vi "Ethernet IP Custom Device Main Page.vi"(8 "error in (no error)":errorcluster, 11 "Node Ptr":T1 format="%.0x") -> (0 "error out":errorcluster)   [LabVIEW 2023, in "Ethernet IP Custom Device Custom Device.lvlib"]
uses:
  Ethernet IP Custom Device Custom Device.lvlib
  <vilib>/NI VeriStand/Custom Device API/Custom Device Item Ref.ctl
  <vilib>/NI VeriStand/Custom Device API/Custom Device Channel.ctl
  <vilib>/NI VeriStand/Custom Device API/Custom Device Channel Type.ctl
  Ethernet IP Global Strings.vi
  <vilib>/NI VeriStand/Custom Device API/Get Item Property (Path).vi
  <vilib>/NI VeriStand/Custom Device API/Get Item Property (I32).vi
  <vilib>/NI VeriStand/Custom Device API/Get Item Property (String).vi
  <vilib>/NI VeriStand/Custom Device API/Set Item Property (String).vi
  <vilib>/NI VeriStand/Custom Device API/Set Item Property (Path).vi
  Ethernet IP Global GUIDs.vi
  <vilib>/NI VeriStand/Custom Device API/Set Item Property (I32).vi
  <vilib>/NI VeriStand/Custom Device API/Custom Device API.lvlib
panel:
  in  "Import Assembly File":bool
  in  "Path to Assembly Import file":path
  in  "Import Selected File":bool
  in  "Path to L5K file":path
  in  "Update Rate (ms)":i32
  in  "Communication Timeout (ms)":i32
  in  "Logix Slot":u16
  in  "Backplane Port":u16
  in  "PLC Address (IP Address)":string
  in  "Header":cluster{"Section Name":string}={"Section Name"="Custom Device Item Settings"}
  in  "Description":string
  in  "Name":string
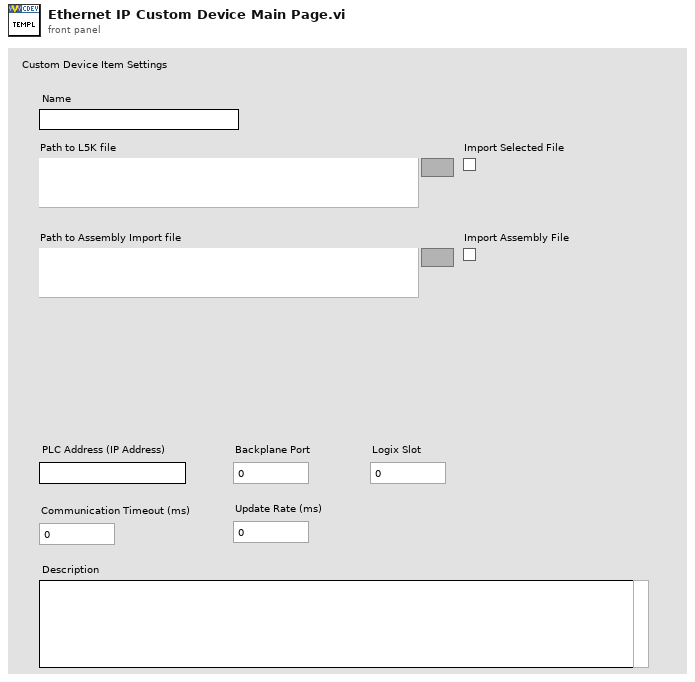
[diagram p1: front panel]
types:
  T1 = typedef "Custom Device API.lvlib/Custom Device Item Ref.ctl" = u64
  T2 = enum8{"Enabled", "Disabled", "Disabled and Grayed Out"}
  T3 = typedef "Custom Device API.lvlib/Custom Device Item Info.ctl" = cluster{"Name":string, "Is Channel":bool, "GUID":string, "Is Waveform":bool}
  T4 = typedef "Custom Device API.lvlib/Custom Device Channel.ctl" = cluster{"Type":T5, "Units":string, "Default Value":dbl, "Faultable":bool, "Scalable":bool}
  T5 = typedef "Custom Device API.lvlib/Custom Device Channel Type.ctl" = enum16{"Input", "Output"}
  T6 = typedef "Custom Device API.lvlib/Custom Device Commands.ctl" = enum16{"Default", "Item renamed", "Shutdown", "Dynamic button pressed"}
  T7 = typedef "Ethernet IP Custom Device Custom Device.lvlib/L5K Internal Data.ctl" = cluster{"L5K Entire String":string, "L5K Extractred String Array":string[], "IP address from CommPath":string, "Configured Tags":T8[], "Data String Array":string[], "Unconfigured Tags":T8[], "# Tags":i32}
  T8 = typedef "Ethernet IP Custom Device Custom Device.lvlib/L5K Tag.ctl" = cluster{"Tag Name":string, "Data Type":T9, "Data Type String":string, "Array Size":i32, "Description":string, "Input?":bool, "Channel Name":string}
  T9 = typedef "Ethernet IP Custom Device Custom Device.lvlib/L5K Data Types.ctl" = enum16{"SINT", "INT", "DINT", "REAL", "BOOL"}
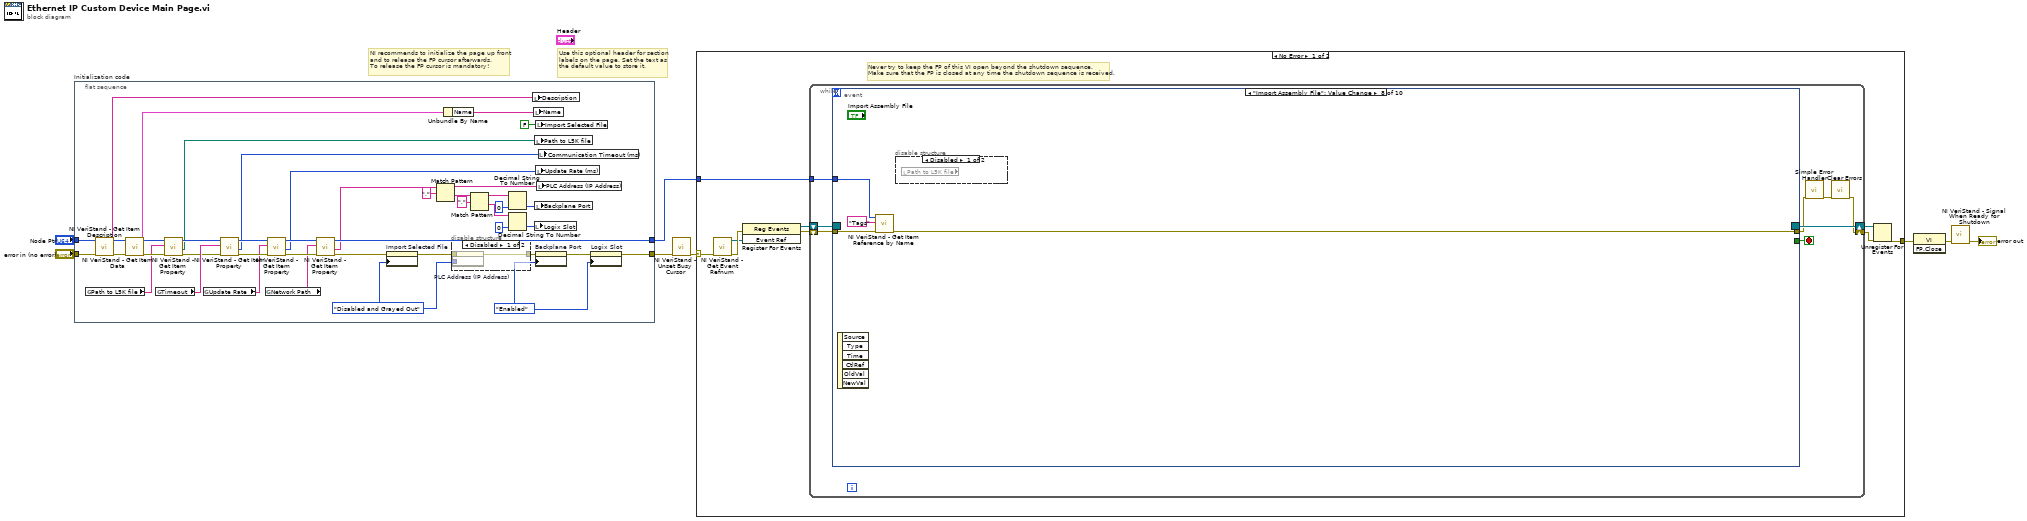
[diagram p0: block diagram]
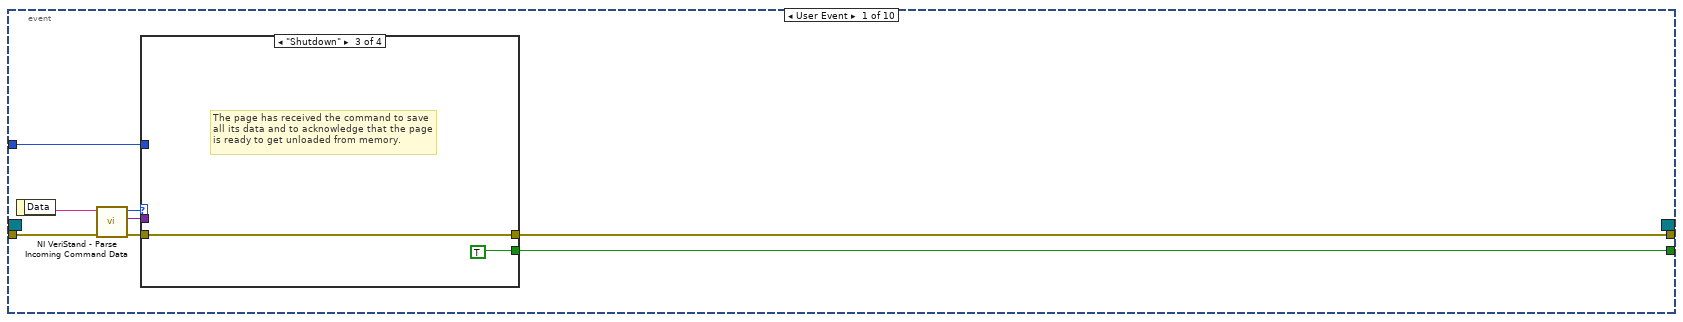
[diagram p2: hidden frame]
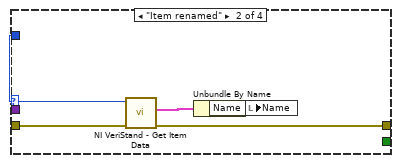
[diagram p4: hidden frame]
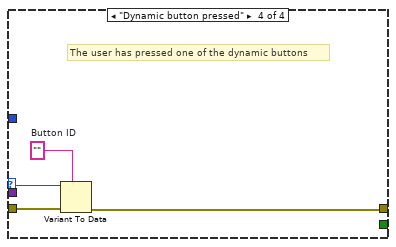
[diagram p5: hidden frame]
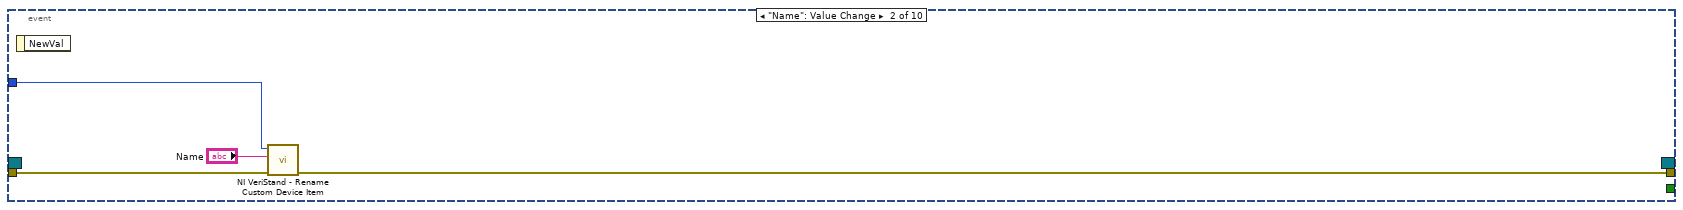
[diagram p6: hidden frame]
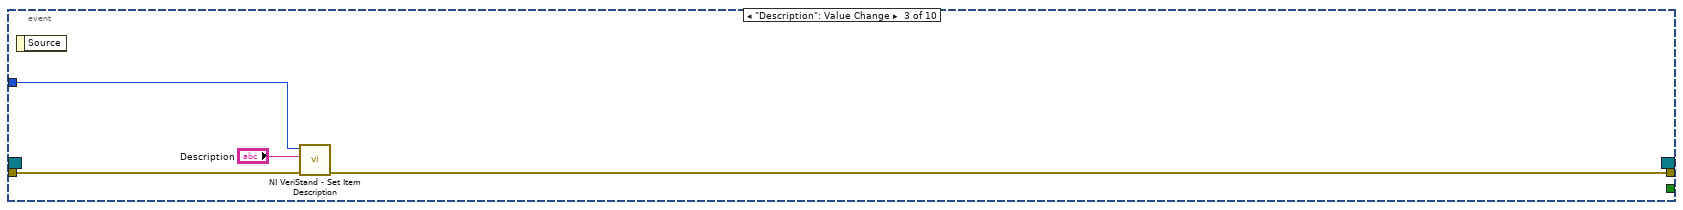
[diagram p7: hidden frame]
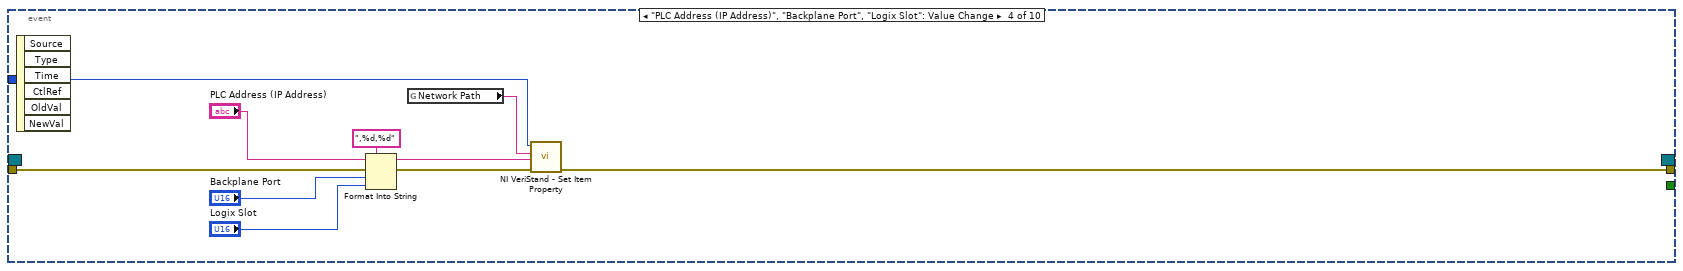
[diagram p8: hidden frame]
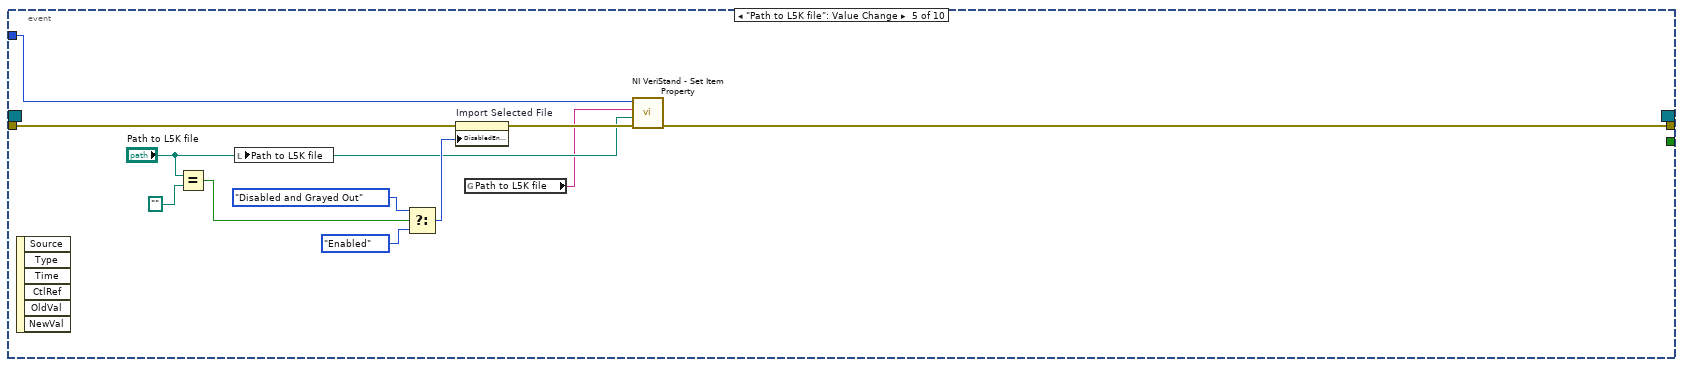
[diagram p9: hidden frame]
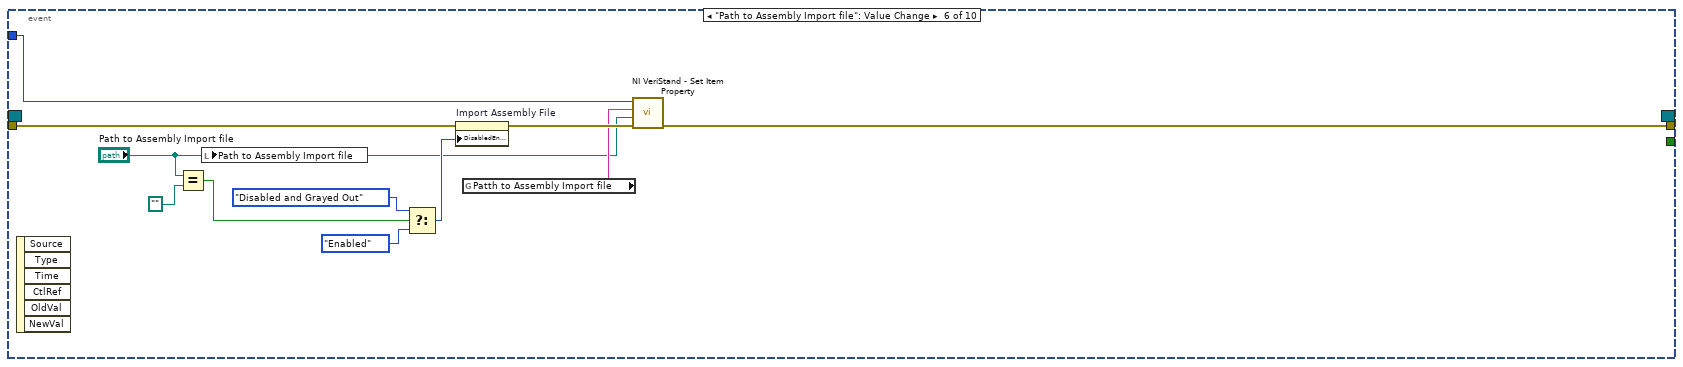
[diagram p10: hidden frame]
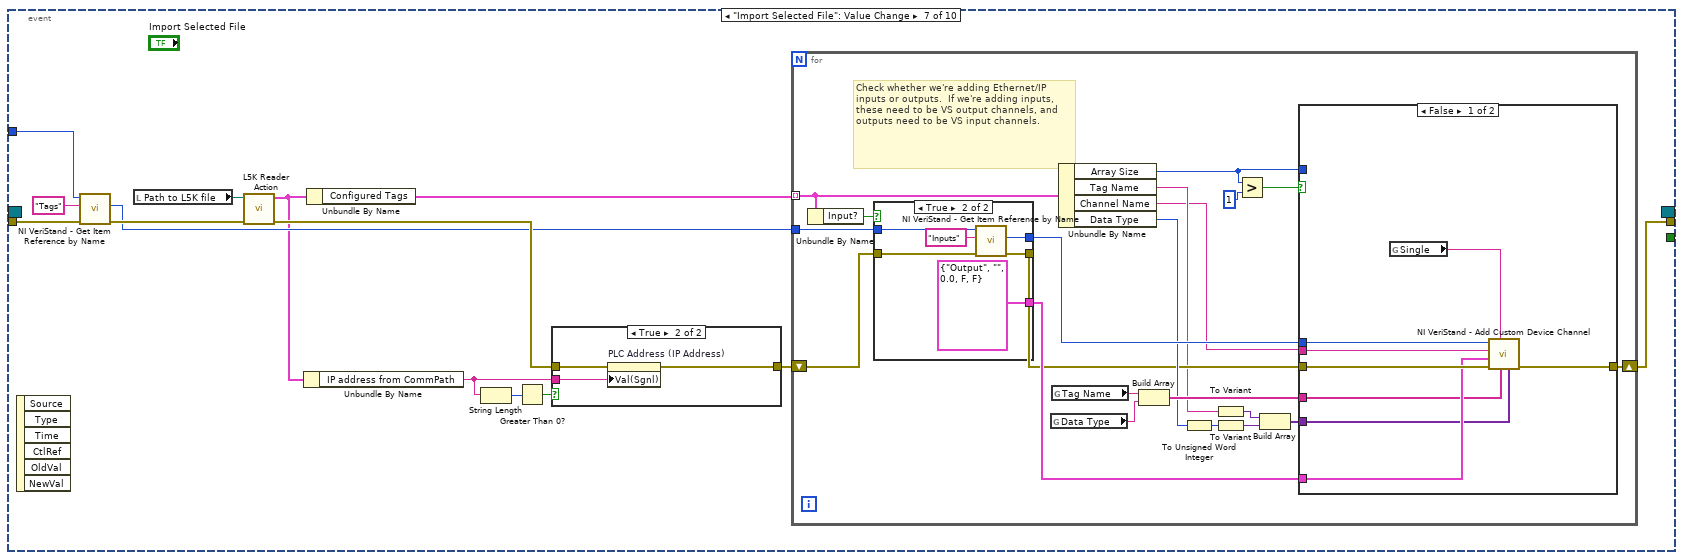
[diagram p11: hidden frame]
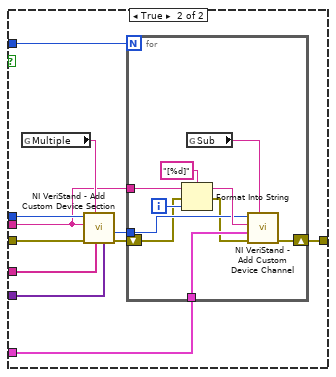
[diagram p12: hidden frame]
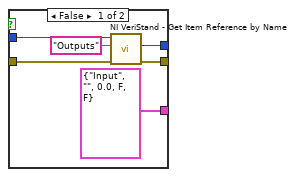
[diagram p13: hidden frame]
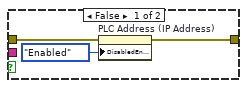
[diagram p14: hidden frame]
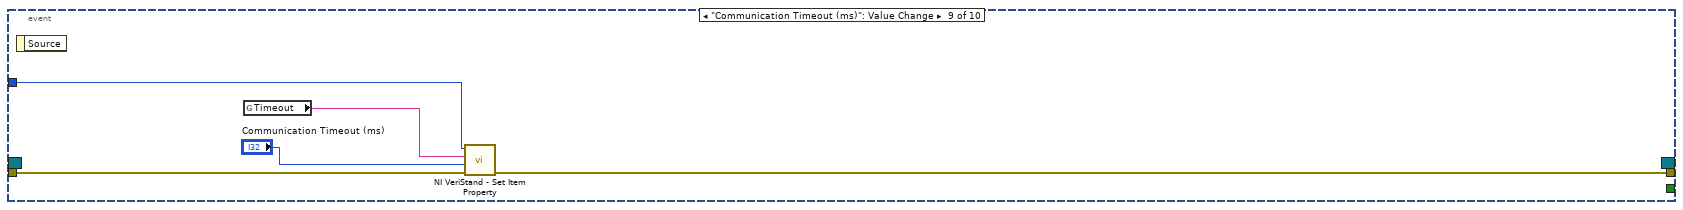
[diagram p16: hidden frame]
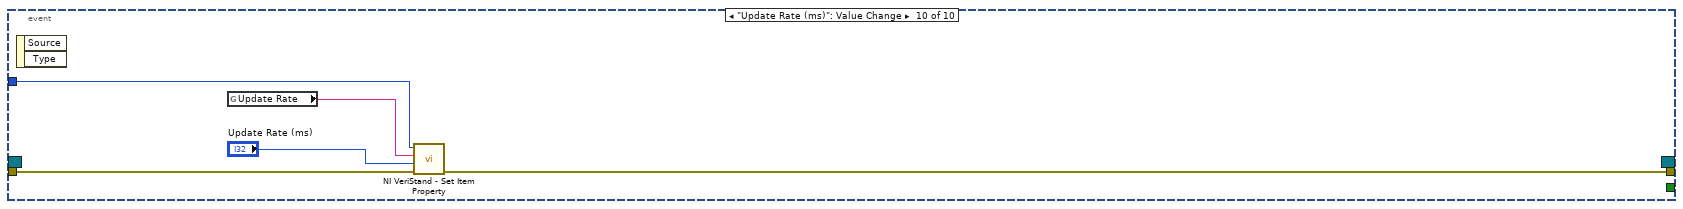
[diagram p17: hidden frame]
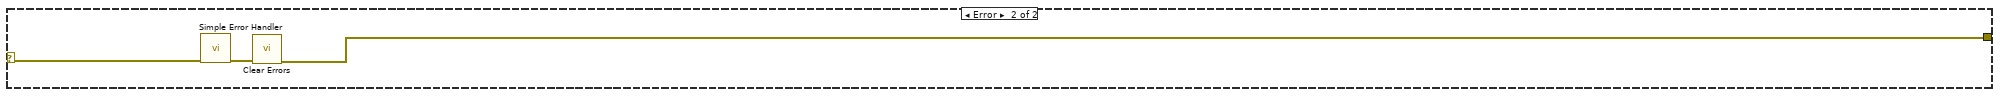
[diagram p18: hidden frame]
diagram:
  # "Use this optional header for section labels on the page. Set the text as the default value to store it."
  # "NI recommends to initialize the page up front\nand to release the FP cursor afterwards.\nTo release the FP cursor is mandatory!"
  n1 = flat-sequence "Initialization code" {
    tunnel: "error in (no error)" -> [w49]
    tunnel: "Node Ptr" -> [w48]
    tunnel: [w20] -> w4
    tunnel: [w27] -> w1
    frame #0 {
      w19 = T2."Enabled" ("Disabled")
      w16 = T2."Disabled and Grayed Out" ("Disabled")
      n2 = global read "Ethernet IP Global Strings.vi" "Path to L5K file"() -> (w10:string)
      n3 = call <vilib>:"NI VeriStand - Get Item Description.vi"("error in (no error)"=w49, "Item Ref in"=w48) -> ("error out"=w46:errorcluster, "Description"=w47:string, "Item Ref out"=w50:T1)  [unwired: 7 out]
      n4 = call <vilib>:"NI VeriStand - Get Item Data.vi"("error in (no error)"=w46, "Item Ref in"=w50) -> ("error out"=w13:errorcluster, "Item Info"=w45:T3, "Item Ref out"=w15:T1)  [unwired: 7 out]
      n5 = global read "Ethernet IP Global Strings.vi" "Timeout"() -> (w33:string)
      n6 = call-poly <vilib>:"NI VeriStand - Get Item Property.vi"("error in (no error)"=w13, "Property Name"=w10, "Item Ref in"=w15) -> ("error out"=w12:errorcluster, "Value"=w9:path, "Item Ref out"=w14:T1)  [unwired: 5 in, 1 out]
      n7 = global read "Ethernet IP Global Strings.vi" "Update Rate"() -> (w32:string)
      n8 = call-poly <vilib>:"NI VeriStand - Get Item Property.vi"("error in (no error)"=w12, "Property Name"=w33, "Item Ref in"=w14) -> ("error out"=w41:errorcluster, "Value"=w30:i32, "Item Ref out"=w43:T1)  [unwired: 5 in, 1 out]
      n9 = global read "Ethernet IP Global Strings.vi" "Network Path"() -> (w31:string)
      n10 = call-poly <vilib>:"NI VeriStand - Get Item Property.vi"("error in (no error)"=w41, "Property Name"=w32, "Item Ref in"=w43) -> ("error out"=w40:errorcluster, "Value"=w28:i32, "Item Ref out"=w42:T1)  [unwired: 5 in, 1 out]
      n11 = call-poly <vilib>:"NI VeriStand - Get Item Property.vi"("error in (no error)"=w40, "Property Name"=w31, "Item Ref in"=w42) -> ("error out"=w18:errorcluster, "Value"=w24:string, "Item Ref out"=w27:T1)  [unwired: 5 in, 1 out]
      n12 = property on="Import Selected File" class="Bool (strict)"(error in=w18, "DisabledEnum"=w16) -> (error out=w17:errorcluster)  [unwired: 1 in, 1 out]
      n13 = Match Pattern(string=w24, regular expression=",") -> (before substring=w25:string, after substring=w23:string)  [unwired: 1 in, 2 out]
      n14 = Unbundle By Name(w45) -> ("Name"=w44:string)
      n15 = disable-structure shown="Disabled" {
        disable-tunnel: [w53 w54] -> w22
        disable-tunnel: w17 -> [w52 w54]
        disable-tunnel: w16 -> [w51 _]
        frame Disabled {
          n16 = property on="PLC Address (IP Address)" class="Str"(error in=w52, "DisabledEnum"=w51) -> (error out=w53:errorcluster)  [unwired: 1 in, 1 out]
        }
        frame Enabled {
        }
      }
      n17 = Match Pattern(string=w23, regular expression=",") -> (before substring=w37:string, after substring=w36:string)  [unwired: 1 in, 2 out]
      n18 = Decimal String To Number(string=w37, default (0L)=u16 0 ("default (0 I32)")) -> (number=w34:u16)  [unwired: 1 in, 1 out]
      n19 = Decimal String To Number(string=w36, default (0L)=u16 0 ("default (0 I32)")) -> (number=w29:u16)  [unwired: 1 in, 1 out]
      n20 = local write "Description"(w47) -> ()
      n21 = local write "Name"(w44) -> ()
      n22 = local write "Logix Slot"(w29) -> ()
      n23 = local write "Path to L5K file"(w9) -> ()
      n24 = local write "Backplane Port"(w34) -> ()
      n25 = local write "Import Selected File"(FALSE ("Import Selected File")) -> ()
      n26 = local write "Update Rate (ms)"(w28) -> ()
      n27 = property on="Backplane Port" class="DigNum (strict)"(error in=w22, "DisabledEnum"=w19) -> (error out=w21:errorcluster)  [unwired: 1 in, 1 out]
      n28 = local write "PLC Address (IP Address)"(w25) -> ()
      n29 = local write "Communication Timeout (ms)"(w30) -> ()
      n30 = property on="Logix Slot" class="DigNum (strict)"(error in=w21, "DisabledEnum"=w19) -> (error out=w20:errorcluster)  [unwired: 1 in, 1 out]
    }
  }
  n31 = call <vilib>:"NI VeriStand - Unset Busy Cursor.vi"("error in (no error)"=w4) -> ("error out"=w3:errorcluster)  [unwired: 10 out]
  n32 = case shown="No Error" w3 {
    selector: w3 -> [w55 w230]
    tunnel: [w60 w228] -> w8
    tunnel: w1 -> [w56 _]
    frame No Error {
      # "Never try to keep the FP of this VI open beyond the shutdown sequence.\nMake sure that the FP is closed at any time the shutdown sequence is received."
      n33 = call <vilib>:"NI VeriStand - Get Event Refnum.vi"("error in (no error)"=w55) -> ("error out"=w63:errorcluster, "Event Ref"=w59:refnum<user-event>)  [unwired: 9 out]
      n34 = register-events(error in=w63, w59) -> (reference out=w57:refnum<event-registration>, error out=w58:errorcluster)  [unwired: 1 in]
      n35 = while {
        tunnel: w56 -> [w67]
        shift-right: [w64] -> w61
        shift-left: w58 -> [w70]
        shift-right: [w71] -> w62
        shift-left: w57 -> [w69]
        stop <- w68 stop-if-true
        n36 = event shown="[7] \"Import Assembly File\": Value Change" {
          selector: w69 -> [_ _ _ _ _ _ _ _ _ _]
          dyn-events: [_ _ _ _ _ _ _ _ _ _] -> w71
          timeout: _ -> [_ _ _ _ _ _ _ _ _ _]
          tunnel: w70 -> [w79 w95 w98 w105 w115 w126 w137 w216 w219 w225]
          tunnel: [w75 _ _ _ _ _ _ _ _ _] -> w68
          tunnel: [w74 w94 w97 w109 w113 w124 w139 w214 w222 w227] -> w66
          tunnel: w67 -> [w73 w93 w99 w108 w112 w123 w138 w215 w221 w226]
          event User Event {
            n37 = event-data() -> ("Data"=w78:string)  [unwired: 1 out]
            n38 = call <vilib>:"NI VeriStand - Parse Incoming Command Data.vi"("error in (no error)"=w79, "Incoming data"=w78) -> ("error out"=w77:errorcluster, "Outgoing data"=w72:variant, "Action"=w76:T6)  [unwired: 7 out]
            n39 = case shown="\"Shutdown\"" w76 {
              tunnel: w77 -> [w80 w85 w86 w91]
              tunnel: [_ _ TRUE _] -> w75
              tunnel: [w80 w82 w86 w88] -> w74
              tunnel: w73 -> [_ w84 _ _]
              tunnel: w72 -> [_ _ _ w90]
              frame "Default", Default {
              }
              frame "Item renamed" {
                n40 = call <vilib>:"NI VeriStand - Get Item Data.vi"("error in (no error)"=w85, "Item Ref in"=w84) -> ("error out"=w82:errorcluster, "Item Info"=w83:T3)  [unwired: 8 out]
                n41 = Unbundle By Name(w83) -> ("Name"=w81:string)
                n42 = local write "Name"(w81) -> ()
              }
              frame "Shutdown" {
                # "The page has received the command to save all its data and to acknowledge that the page is ready to get unloaded from memory."
              }
              frame "Dynamic button pressed" {
                w89 = ""  # Button ID
                # "The user has pressed one of the dynamic buttons"
                n43 = Variant To Data(error in=w91, type=w89, Variant=w90) -> (error out=w88:errorcluster)  [unwired: 1 out]
              }
            }
          }
          event "Name": Value Change {
            n44 = event-data() -> ()  [unwired: 2 out]
            n45 = call <vilib>:"NI VeriStand - Rename Custom Device Item.vi"("error in (no error)"=w95, "New Name"="Name", "Item Ref in"=w93) -> ("error out"=w94:errorcluster)  [unwired: 1 in, 7 out]
          }
          event "Description": Value Change {
            n46 = event-data() -> ()  [unwired: 2 out]
            n47 = call <vilib>:"NI VeriStand - Set Item Description.vi"("error in (no error)"=w98, "Description"="Description", "Item Ref in"=w99) -> ("error out"=w97:errorcluster)  [unwired: 8 out]
          }
          event "PLC Address (IP Address)", "Backplane Port", "Logix Slot": Value Change {
            n48 = event-data() -> ()  [unwired: 7 out]
            n49 = Format Into String(format string=",%d,%d", initial string="PLC Address (IP Address)", error in=w105, "Backplane Port", "Logix Slot") -> (resulting string=w103:string, error out=w104:errorcluster)
            n50 = global read "Ethernet IP Global Strings.vi" "Network Path"() -> (w107:string)
            n51 = call-poly <vilib>:"NI VeriStand - Set Item Property.vi"("error in (no error)"=w104, "Value"=w103, "Property Name"=w107, "Item Ref in"=w108) -> ("error out"=w109:errorcluster)  [unwired: 5 in, 2 out]
          }
          event "Path to L5K file": Value Change {
            n52 = event-data() -> ()  [unwired: 7 out]
            n53 = Equal?(x="Path to L5K file", y=path "") -> (x = y?=w119:bool)
            n54 = local write "Path to L5K file"("Path to L5K file") -> ()
            n55 = Select(t=T2."Disabled and Grayed Out" ("Disabled"), s=w119, f=T2."Enabled" ("Disabled")) -> (s? t:f=w116:T2)
            n56 = property on="Import Selected File" class="Bool (strict)"(error in=w115, "DisabledEnum"=w116) -> (error out=w114:errorcluster)  [unwired: 1 in, 1 out]
            n57 = global read "Ethernet IP Global Strings.vi" "Path to L5K file"() -> (w110:string)
            n58 = call-poly <vilib>:"NI VeriStand - Set Item Property.vi"("error in (no error)"=w114, "Value"="Path to L5K file", "Property Name"=w110, "Item Ref in"=w112) -> ("error out"=w113:errorcluster)  [unwired: 5 in, 2 out]
          }
          event "Path to Assembly Import file": Value Change {
            n59 = event-data() -> ()  [unwired: 7 out]
            n60 = Equal?(x="Path to Assembly Import file", y=path "") -> (x = y?=w130:bool)
            n61 = local write "Path to Assembly Import file"("Path to Assembly Import file") -> ()
            n62 = Select(t=T2."Disabled and Grayed Out" ("Disabled"), s=w130, f=T2."Enabled" ("Disabled")) -> (s? t:f=w127:T2)
            n63 = property on="Import Assembly File" class="Bool (strict)"(error in=w126, "DisabledEnum"=w127) -> (error out=w125:errorcluster)  [unwired: 1 in, 1 out]
            n64 = global read "Ethernet IP Global Strings.vi" "Patth to Assembly Import file"() -> (w122:string)
            n65 = call-poly <vilib>:"NI VeriStand - Set Item Property.vi"("error in (no error)"=w125, "Value"="Path to Assembly Import file", "Property Name"=w122, "Item Ref in"=w123) -> ("error out"=w124:errorcluster)  [unwired: 5 in, 2 out]
          }
          event "Import Selected File": Value Change {
            n66 = event-data() -> ()  [unwired: 7 out]
            n67 = call <vilib>:"NI VeriStand - Get Item Reference by Name.vi"("error in (no error)"=w137, "Item Name"="Tags", "Parent Ref in"=w138) -> ("error out"=w135:errorcluster, "Item Ref"=w134:T1)  [unwired: 5 in, 2 out]
            n68 = local read "Path to L5K file"() -> (w132:path)
            n69 = call "L5K Reader Action.vi"("error in"=w135, "L5K File Path"=w132) -> ("error out"=w142:errorcluster, "L5K Information"=w133:T7)  [unwired: 7 in, 1 out]
            n70 = Unbundle By Name(w133) -> ("IP address from CommPath"=w143:string)
            n71 = Unbundle By Name(w133) -> ("Configured Tags"=w141:T8[])
            n72 = String Length(string=w143) -> (length=w145:i32)
            n73 = Greater Than 0?(x=w145) -> (x > 0?=w144:bool)
            n74 = case shown="True" w144 {
              tunnel: w143 -> [_ w213]
              tunnel: w142 -> [w209 w212]
              tunnel: [w208 w211] -> w140
              frame False {
                n75 = property on="PLC Address (IP Address)" class="Str"(error in=w209, "DisabledEnum"=T2."Enabled" ("Disabled")) -> (error out=w208:errorcluster)  [unwired: 1 in, 1 out]
              }
              frame True {
                n76 = property on="PLC Address (IP Address)" class="Str"(error in=w212, "Val(Sgnl)"=w213) -> (error out=w211:errorcluster)  [unwired: 1 in, 1 out]
              }
            }
            n77 = for {
              tunnel: w134 -> [w156]
              shift-right: [w154] -> w139
              shift-left: w140 -> [w149]
              tunnel: w141 -> [w150] mode=indexing
              # "Check whether we're adding Ethernet/IP\ninputs or outputs.  If we're adding inputs,\nthese need to be VS output channels, and\noutputs need to be VS input channels."
              n78 = Unbundle By Name(w150) -> ("Input?"=w153:bool)
              n79 = case shown="True" w153 {
                tunnel: [T4 {"Type"=enum."Input", "Units"="", "Default Value"=0.0, "Faultable"=FALSE, "Scalable"=FALSE} ("Channel") T4 {"Type"=enum."Output", "Units"="", "Default Value"=0.0, "Faultable"=FALSE, "Scalable"=FALSE} ("Channel")] -> w166
                tunnel: w156 -> [w200 w206]
                tunnel: [w198 w205] -> w155
                tunnel: w149 -> [w197 w203]
                tunnel: [w196 w202] -> w148
                frame False {
                  n80 = call <vilib>:"NI VeriStand - Get Item Reference by Name.vi"("error in (no error)"=w197, "Item Name"="Outputs", "Parent Ref in"=w200) -> ("error out"=w196:errorcluster, "Item Ref"=w198:T1)  [unwired: 5 in, 2 out]
                }
                frame True {
                  n81 = call <vilib>:"NI VeriStand - Get Item Reference by Name.vi"("error in (no error)"=w203, "Item Name"="Inputs", "Parent Ref in"=w206) -> ("error out"=w202:errorcluster, "Item Ref"=w205:T1)  [unwired: 5 in, 2 out]
                }
              }
              n82 = global read "Ethernet IP Global Strings.vi" "Data Type"() -> (w157:string)
              n83 = global read "Ethernet IP Global Strings.vi" "Tag Name"() -> (w158:string)
              n84 = Unbundle By Name(w150) -> ("Array Size"=w151:i32, "Tag Name"=w147:string, "Channel Name"=w146:string, "Data Type"=w152:T9)
              n85 = Build Array(w158, w157) -> (w161:string[])
              n86 = To Unsigned Word Integer(number=w152) -> (unsigned 16bit integer=w160:u16)
              n87 = To Variant(anything=w147) -> (Variant=w159:variant)
              n88 = To Variant(anything=w160) -> (Variant=w163:variant)
              n89 = Greater?(x=w151, y=1) -> (0:w164:bool)
              n90 = Build Array(w159, w163) -> (w162:variant[])
              n91 = case shown="False" w164 {
                tunnel: w148 -> [w174 w183]
                tunnel: w166 -> [w173 w175]
                tunnel: w146 -> [w167 w177]
                tunnel: w162 -> [w171 w185]
                tunnel: w161 -> [w172 w184]
                tunnel: w155 -> [w170 w180]
                tunnel: [w168 w178] -> w154
                tunnel: w151 -> [_ w176]
                frame False {
                  n92 = global read "Ethernet IP Global GUIDs.vi" "Single"() -> (w169:string)
                  n93 = call <vilib>:"NI VeriStand - Add Custom Device Channel.vi"("Property Values"=w171, "Property names"=w172, "GUID (Default Channel)"=w169, "error in (no error)"=w174, "Channel"=w173, "Channel Name"=w167, "Parent Ref in"=w170) -> ("error out"=w168:errorcluster)  [unwired: 1 in, 3 out]
                }
                frame True {
                  n94 = global read "Ethernet IP Global GUIDs.vi" "Multiple"() -> (w179:string)
                  n95 = call <vilib>:"NI VeriStand - Add Custom Device Section.vi"("Property Values"=w185, "Property names"=w184, "GUID (Default Section)"=w179, "error in (no error)"=w183, "Section Name"=w177, "Parent Ref in"=w180) -> ("error out"=w181:errorcluster, "Section Ptr"=w182:T1)  [unwired: 2 in, 2 out]
                  n96 = for {
                    N: w176 -> [_]
                    tunnel: w182 -> [w192]
                    tunnel: w175 -> [w191]
                    shift-right: [w189] -> w178
                    shift-left: w181 -> [w187]
                    tunnel: w177 -> [w188]
                    i -> [w195]
                    n97 = Format Into String(format string="[%d]", initial string=w188, error in=w187, w195) -> (resulting string=w193:string, error out=w186:errorcluster)
                    n98 = global read "Ethernet IP Global GUIDs.vi" "Sub"() -> (w190:string)
                    n99 = call <vilib>:"NI VeriStand - Add Custom Device Channel.vi"("GUID (Default Channel)"=w190, "error in (no error)"=w186, "Channel"=w191, "Channel Name"=w193, "Parent Ref in"=w192) -> ("error out"=w189:errorcluster)  [unwired: 3 in, 3 out]
                  }
                }
              }
            }
          }
          event "Import Assembly File": Value Change {
            n100 = event-data() -> ()  [unwired: 7 out]
            n101 = call <vilib>:"NI VeriStand - Get Item Reference by Name.vi"("error in (no error)"=w216, "Item Name"="Tags", "Parent Ref in"=w215) -> ("error out"=w214:errorcluster)  [unwired: 5 in, 3 out]
            n102 = disable-structure shown="Disabled" {
              frame Disabled {
                n103 = local read "Path to L5K file"() -> ()  [unwired: 1 out]
              }
              frame Enabled {
              }
            }
          }
          event "Communication Timeout (ms)": Value Change {
            n104 = event-data() -> ()  [unwired: 2 out]
            n105 = global read "Ethernet IP Global Strings.vi" "Timeout"() -> (w220:string)
            n106 = call-poly <vilib>:"NI VeriStand - Set Item Property.vi"("error in (no error)"=w219, "Value"="Communication Timeout (ms)", "Property Name"=w220, "Item Ref in"=w221) -> ("error out"=w222:errorcluster)  [unwired: 5 in, 2 out]
          }
          event "Update Rate (ms)": Value Change {
            n107 = event-data() -> ()  [unwired: 3 out]
            n108 = global read "Ethernet IP Global Strings.vi" "Update Rate"() -> (w224:string)
            n109 = call-poly <vilib>:"NI VeriStand - Set Item Property.vi"("error in (no error)"=w225, "Value"="Update Rate (ms)", "Property Name"=w224, "Item Ref in"=w226) -> ("error out"=w227:errorcluster)  [unwired: 5 in, 2 out]
          }
        }
        n110 = call <vilib>:"Simple Error Handler.vi"("error in (no error)"=w66) -> ("error out"=w65:errorcluster)  [unwired: 1 in, 7 out]
        n111 = call <vilib>:"Clear Errors.vi"("error in (no error)"=w65) -> ("error out"=w64:errorcluster)  [unwired: 1 in, 5 out]
      }
      n112 = Unregister For Events(event registration refnum=w62, error in=w61) -> (error out=w60:errorcluster)
    }
    frame Error {
      n113 = call <vilib>:"Simple Error Handler.vi"("error in (no error)"=w230) -> ("error out"=w229:errorcluster)  [unwired: 1 in, 7 out]
      n114 = call <vilib>:"Clear Errors.vi"("error in (no error)"=w229) -> ("error out"=w228:errorcluster)  [unwired: 1 in, 5 out]
    }
  }
  n115 = invoke class="VI" method="FP.Close"(error in=w8) -> (error out=w7:errorcluster)  [unwired: 2 in, 2 out]
  n116 = call <vilib>:"NI VeriStand - Signal When Ready for Shutdown.vi"("error in (no error)"=w7) -> ("error out"=→"error out":errorcluster)  [unwired: 10 out]
